vi "Get_Blocking_Complete.vi"(0 "Update Functions In":cluster{string, string[], dbl[], dbl}[](array[cluster])) -> (1 "Update Functions Out":cluster{string, string[], dbl[], dbl}[](array[cluster]), 2 "Event Completed":bool)   [LabVIEW 2011]
doc: "This VI takes the array of update functions as its input, and determines if any currently blocking API functions are complete, necessitating a continuation of the growth sequence."
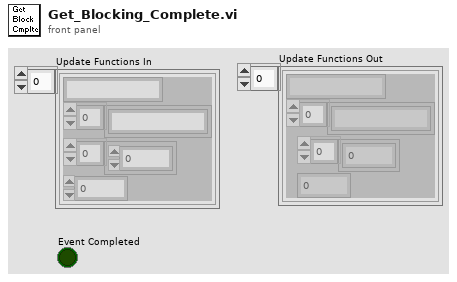
[diagram p1: front panel]
types:
  T1 = cluster{string, "Argument List Out":string[], dbl[], dbl}
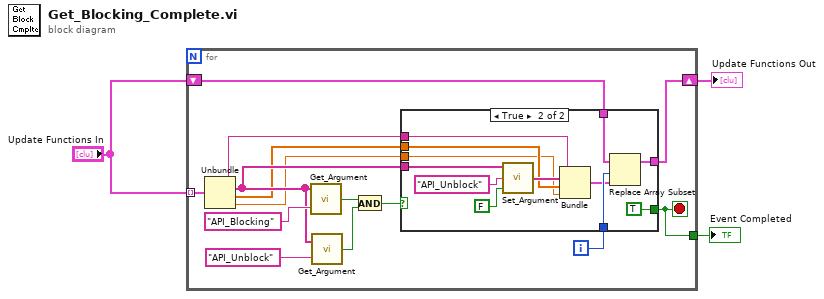
[diagram p0: block diagram]
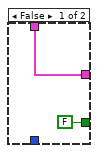
[diagram p2: hidden frame]
diagram:
  n1 = for {
    shift-right: [w5] -> w3
    shift-left: "Update Functions In" -> [w6]
    tunnel: "Update Functions In" -> [w17] mode=indexing
    tunnel: [w4] -> w1
    i -> [w7]
    stop <- w4 stop-if-true
    n2 = Unbundle(w17) -> (w10:string, w11:string[], w9:dbl[], w8:dbl)
    n3 = call "Get_Argument.vi"("Argument"="API_Blocking", "Argument List"=w11) -> ("Enabled"=w14:bool)
    n4 = call "Get_Argument.vi"("Argument"="API_Unblock", "Argument List"=w11) -> ("Enabled"=w13:bool)
    n5 = And(x=w14, y=w13) -> (x .and. y?=w12:bool)
    n6 = case shown="True" w12 {
      tunnel: w11 -> [_ w31]
      tunnel: w10 -> [_ w27]
      tunnel: w9 -> [_ w26]
      tunnel: w8 -> [_ w25]
      tunnel: w7 -> [_ w24]
      tunnel: w6 -> [w19 w22]
      tunnel: [w19 w21] -> w5
      tunnel: [FALSE TRUE] -> w4
      frame False {
      }
      frame True {
        n7 = call "Set_Argument.vi"("Enable"=FALSE, "Argument"="API_Unblock", "Argument List In"=w31) -> ("Argument List Out"=w28:string[])
        n8 = Bundle(w27, "Argument List Out"=w28, w26, w25) -> (w23:T1)  [unwired: 1 in]
        n9 = Replace Array Subset(array=w22, new element=w23, index=w24) -> (w21:cluster{string, string[], dbl[], dbl}[])
      }
    }
  }
  "Update Functions Out" <- w3
  "Event Completed" <- w1
